vi "Read Contour Display Rate (SubVI).vi"() -> (3 "Rate (Hz)":u32)   [LabVIEW 2020]
uses:
  <vilib>/Utility/config.llb/Read Key (U32).vi
  <vilib>/Utility/config.llb/Write Key (U32).vi
  <vilib>/Utility/config.llb/NI_LVConfig.lvlib
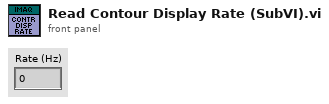
[diagram p1: front panel]
types:
  T1 = typedef "NI_LVConfig.lvlib/Config Data RefNum.ctl" = refnum<k1>
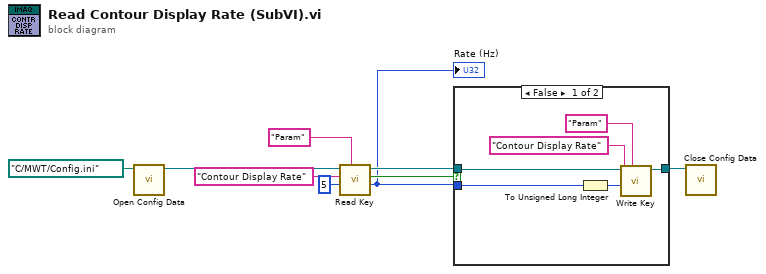
[diagram p0: block diagram]
diagram:
  n1 = call <vilib>:"Open Config Data.vi"("configuration file path"=path "C:/MWT/Config.ini") -> ("refnum"=w6:T1)  [unwired: 8 in, 2 out]
  n2 = call-poly <vilib>:"Read Key.vi"("section"="Param", "default value"=u32 5, "key"="Contour Display Rate" ("section"), "refnum"=w6) -> ("value"=w1:u32, "found?"=w4:bool, "refnum out"=w3:T1)  [unwired: 4 in, 1 out]
  "Rate (Hz)" <- w1
  n3 = case shown="False" w4 {
    tunnel: w3 -> [w12 w16]
    tunnel: [w11 w16] -> w2
    tunnel: w1 -> [w10 _]
    frame False {
      n4 = To Unsigned Long Integer(number=w10) -> (unsigned 32bit integer=w14:u32)
      n5 = call-poly <vilib>:"Write Key.vi"("section"="Param", "value"=w14, "key"="Contour Display Rate" ("section"), "refnum"=w12) -> ("refnum out"=w11:T1)  [unwired: 5 in, 2 out]
    }
    frame True {
    }
  }
  n6 = call <vilib>:"Close Config Data.vi"("refnum"=w2) -> ()  [unwired: 9 in, 2 out]
